vi "toml_token_next.vi"(9 "offset (0)":i32, 11 "json":string) -> (1 "offset past token":i32, 2 "arg":string, 3 "token":T1)   [LabVIEW 2017]
uses:
  toml_token.ctl
  <vilib>/regexp/Match Regular Expression.xnode
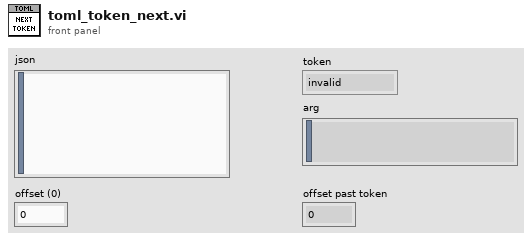
[diagram p1: front panel]
types:
  T1 = typedef "toml_token.ctl" = enum8{"invalid", "bool", "string", "int", "uint", "float", "datetime", "array", "inline_table", "table", "table_element", "key", "comment", "comment_inline", "end"}
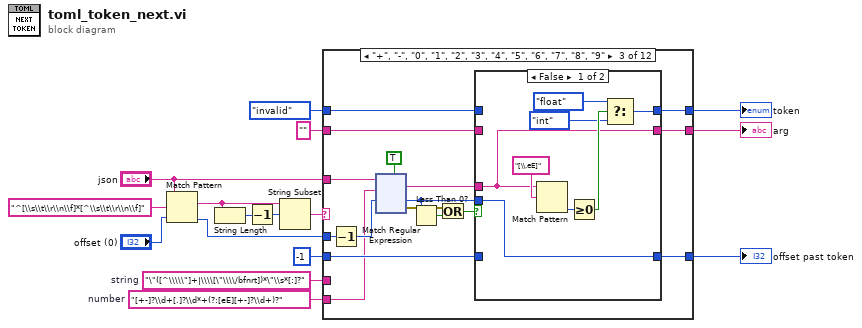
[diagram p0: block diagram]
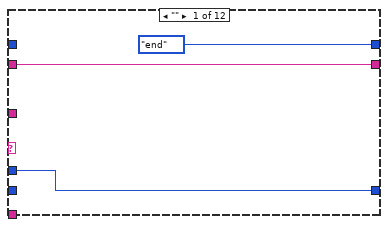
[diagram p2: hidden frame]
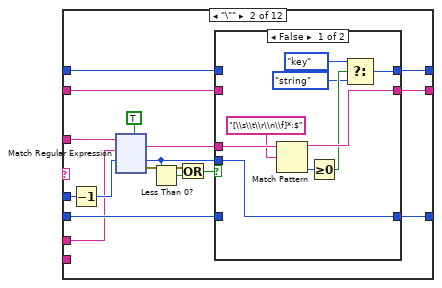
[diagram p3: hidden frame]
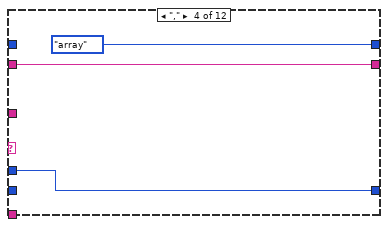
[diagram p6: hidden frame]
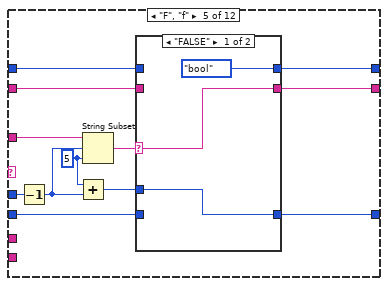
[diagram p7: hidden frame]
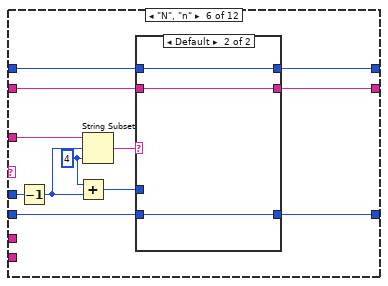
[diagram p9: hidden frame]
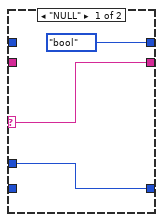
[diagram p10: hidden frame]
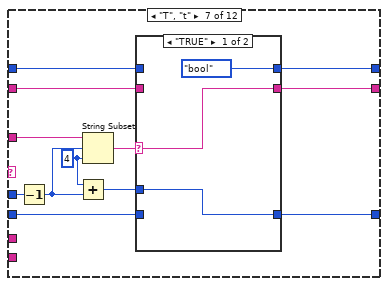
[diagram p11: hidden frame]
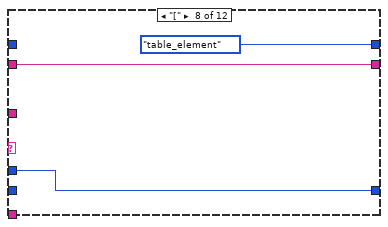
[diagram p13: hidden frame]
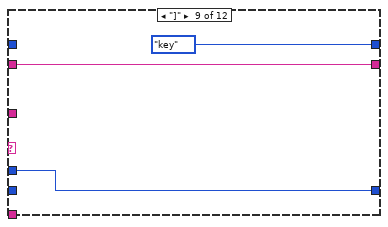
[diagram p14: hidden frame]
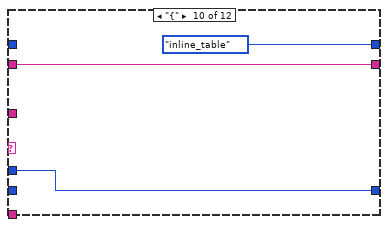
[diagram p15: hidden frame]
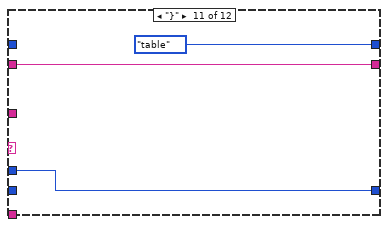
[diagram p16: hidden frame]
diagram:
  w1 = "[+-]?\\d+[.]?\\d*+(?:[eE][+-]?\\d+)?"  # number
  w2 = "\"([^\\\\\"]+|\\\\[\"\\\\/bfnrt])*\"\\s*[:]?"  # string
  n1 = Match Pattern(string="json", regular expression="^[\\s\\t\\r\\n\\f]*[^\\s\\t\\r\\n\\f]", offset (0)="offset (0)") -> (match substring=w13:string, offset past match=w8:i32)  [unwired: 2 out]
  n2 = String Length(string=w13) -> (length=w14:i32)
  n3 = Decrement(x=w14) -> (x-1=w12:i32)
  n4 = String Subset(string=w13, offset (0)=w12) -> (substring=w11:string)  [unwired: 1 in]
  n5 = case shown="\"+\", \"-\", \"0\", \"1\", \"2\", \"3\", \"4\", \"5\", \"6\", \"7\", \"8\", \"9\"" w11 {
    tunnel: [toml_token."end" ("token") w24 w166 toml_token."array" ("token") w307 w325 w343 toml_token."table_element" ("token") toml_token."key" ("token") toml_token."inline_table" ("token") toml_token."table" ("token") w374] -> w10
    tunnel: toml_token."invalid" ("token") -> [_ w23 w165 _ w306 w324 w342 _ _ _ _ w374]
    tunnel: w8 -> [w18 w33 w175 w304 w316 w334 w352 w361 w364 w367 w370 _]
    tunnel: [w18 w28 w170 w304 w311 w329 w347 w361 w364 w367 w370 w373] -> w7
    tunnel: -1 ("offset past match") -> [_ w27 w169 _ w310 w328 w346 _ _ _ _ w373]
    tunnel: [w19 w26 w168 w305 w309 w327 w345 w362 w365 w368 w371 w372] -> w5
    tunnel: "" -> [w19 w25 w167 w305 w308 w326 w344 w362 w365 w368 w371 w372]
    tunnel: "json" -> [_ w35 w177 _ w317 w335 w353 _ _ _ _ _]
    tunnel: w2 -> [_ w20 _ _ _ _ _ _ _ _ _ _]
    tunnel: w1 -> [_ _ w162 _ _ _ _ _ _ _ _ _]
    frame "" {
    }
    frame "\"" {
      n6 = Decrement(x=w33) -> (x-1=w32:i32)
      n7 = xnode "Match Regular Expression"("input string"=w35, "regular expression"=w20, "offset (0)"=w32, "multiline? (F)"=TRUE) -> ("whole match"=w21:string, "offset past match"=w22:i32, "error out"=w31:errorcluster)  [unwired: 2 in, 2 out]
      n8 = Less Than 0?(x=w22) -> (x < 0?=w30:bool)
      n9 = Or(x=w31, y=w30) -> (x .or. y?=w29:bool)
      n10 = case shown="False" w29 {
        tunnel: [w38 w47] -> w28
        tunnel: w27 -> [_ w47]
        tunnel: [w42 w46] -> w26
        tunnel: w25 -> [_ w46]
        tunnel: [w39 w45] -> w24
        tunnel: w23 -> [_ w45]
        tunnel: w22 -> [w38 _]
        tunnel: w21 -> [w44 _]
        frame False {
          n11 = Match Pattern(string=w44, regular expression="[\\s\\t\\r\\n\\f]*:$") -> (before substring=w42:string, offset past match=w41:i32)  [unwired: 1 in, 2 out]
          n12 = Greater Or Equal To 0?(x=w41) -> (x >= 0?=w40:bool)
          n13 = Select(t=toml_token."key" ("token"), s=w40, f=toml_token."string" ("token")) -> (s? t:f=w39:T1)
        }
        frame True {
        }
      }
    }
    frame "+", "-", "0", "1", "2", "3", "4", "5", "6", "7", "8", "9" {
      n14 = Decrement(x=w175) -> (x-1=w174:i32)
      n15 = xnode "Match Regular Expression"("input string"=w177, "regular expression"=w162, "offset (0)"=w174, "multiline? (F)"=TRUE) -> ("whole match"=w163:string, "offset past match"=w164:i32, "error out"=w173:errorcluster)  [unwired: 2 in, 2 out]
      n16 = Less Than 0?(x=w164) -> (x < 0?=w172:bool)
      n17 = Or(x=w173, y=w172) -> (x .or. y?=w171:bool)
      n18 = case shown="False" w171 {
        tunnel: [w181 w188] -> w170
        tunnel: w169 -> [_ w188]
        tunnel: [w180 w187] -> w168
        tunnel: w167 -> [_ w187]
        tunnel: [w182 w186] -> w166
        tunnel: w165 -> [_ w186]
        tunnel: w164 -> [w181 _]
        tunnel: w163 -> [w180 _]
        frame False {
          n19 = Match Pattern(string=w180, regular expression="[\\.eE]") -> (offset past match=w184:i32)  [unwired: 1 in, 3 out]
          n20 = Greater Or Equal To 0?(x=w184) -> (x >= 0?=w183:bool)
          n21 = Select(t=toml_token."float" ("token"), s=w183, f=toml_token."int" ("token")) -> (s? t:f=w182:T1)
        }
        frame True {
        }
      }
    }
    frame "," {
    }
    frame "F", "f" {
      w314 = 5 ("length (rest)")
      n22 = Decrement(x=w316) -> (x-1=w315:i32)
      n23 = Add(x=w314, y=w315) -> (x+y=w313:i32)
      n24 = String Subset(string=w317, offset (0)=w315, length (rest)=w314) -> (substring=w312:string)
      n25 = case shown="\"FALSE\"" w312 {
        selector: w312 -> [w320 _]
        tunnel: w313 -> [w319 _]
        tunnel: [w319 w323] -> w311
        tunnel: w310 -> [_ w323]
        tunnel: [w320 w322] -> w309
        tunnel: w308 -> [_ w322]
        tunnel: [toml_token."bool" ("token") w321] -> w307
        tunnel: w306 -> [_ w321]
        frame "FALSE" {
        }
        frame Default {
        }
      }
    }
    frame "N", "n" {
      w332 = 4 ("length (rest)")
      n26 = Decrement(x=w334) -> (x-1=w333:i32)
      n27 = Add(x=w332, y=w333) -> (x+y=w331:i32)
      n28 = String Subset(string=w335, offset (0)=w333, length (rest)=w332) -> (substring=w330:string)
      n29 = case shown="Default" w330 {
        selector: w330 -> [w338 _]
        tunnel: w331 -> [w337 _]
        tunnel: [w337 w341] -> w329
        tunnel: w328 -> [_ w341]
        tunnel: [w338 w340] -> w327
        tunnel: w326 -> [_ w340]
        tunnel: [toml_token."bool" ("token") w339] -> w325
        tunnel: w324 -> [_ w339]
        frame "NULL" {
        }
        frame Default {
        }
      }
    }
    frame "T", "t" {
      w350 = 4 ("length (rest)")
      n30 = Decrement(x=w352) -> (x-1=w351:i32)
      n31 = Add(x=w350, y=w351) -> (x+y=w349:i32)
      n32 = String Subset(string=w353, offset (0)=w351, length (rest)=w350) -> (substring=w348:string)
      n33 = case shown="\"TRUE\"" w348 {
        selector: w348 -> [w356 _]
        tunnel: w349 -> [w355 _]
        tunnel: [w355 w359] -> w347
        tunnel: w346 -> [_ w359]
        tunnel: [w356 w358] -> w345
        tunnel: w344 -> [_ w358]
        tunnel: [toml_token."bool" ("token") w357] -> w343
        tunnel: w342 -> [_ w357]
        frame "TRUE" {
        }
        frame Default {
        }
      }
    }
    frame "[" {
    }
    frame "]" {
    }
    frame "{" {
    }
    frame "}" {
    }
    frame Default {
    }
  }
  "token" <- w10
  "arg" <- w5
  "offset past token" <- w7
